vi "Handle Command.vi"(8 "error in":errorcluster, 10 "Change Laser Frequency in":refnum<class "Change Laser Frequency.lvclass">, 11 "Object In":refnum<class>) -> (0 "error out":errorcluster, 1 "Command Successful?":bool, 2 "Change Laser Frequency out":refnum<class "Change Laser Frequency.lvclass">, 3 "Object Out":refnum<class>)   [LabVIEW 2018, in "ePAS Library.lvlib" / "Change Laser Frequency.lvclass"]
doc: "Abstract method for accomplishing the execution of a command directed to an instrument object on the wire."
uses:
  Change Laser Frequency.lvclass
  Instrument/ePAS.lvclass
  C:/Users/Labview/Documents/exscalabar_server/reusable/PAS/Main/PAS.lvclass
  C:/Users/Labview/Documents/exscalabar_server/reusable/Instrument/Instrument.lvclass
  reusable/PAS/Data/Main/PAS Data.lvclass
  C:/Users/Labview/Documents/exscalabar_server/reusable/Data/Data.lvclass
  Change Laser Frequency.lvclass/Change Laser Frequency.ctl
  Instrument/ePAS.lvclass/ePAS.ctl
  reusable/Instrument/Instrument.lvclass/Instrument.ctl
  reusable/PAS/Data/Cell/PAS Cell Data.lvclass/PAS Cell Data.ctl
  reusable/PAS/Cell/PAS Cell.lvclass/PAS Cell.ctl
  reusable/PAS/Data/Cell/Write fmod.vi
  reusable/PAS/Cell/Write Mod Freq.vi
  Instrument/Accessors/Read FPGA Session.vi
  reusable/Instrument/Read ExtCom.vi
  reusable/Instrument/Read Log Session.vi
  reusable/Instrument/Read Data.vi
  reusable/Instrument/Write Data.vi
  reusable/PAS/Main/Read Cells.vi
  <vilib>/Utility/error.llb/Error Cluster From Error Code.vi
  <vilib>/rvi/errors/niLvFpgaAdjustHostInterfaceError.vi
  reusable/PAS/Data/Main/Read CellData.vi
  reusable/PAS/Data/Main/Write CellData.vi
  reusable/PAS/Main/Write Cells.vi
  reusable/PAS/Cell/PAS Cell.lvclass
  <userlib>/_Session Fwk/Session - Root.lvclass
  reusable/Data/Data.lvclass
  <vilib>/rvi/interface/nirviReadWriteControl/nirviReadWriteControl.xnode
  FPGA/R FPGA Ref.ctl
  FPGA Bitfiles/FPGAServer.lvbitx
  reusable/PAS/Data/Cell/PAS Cell Data.lvclass
  FPGA/Session/Exscalabar FPGA.lvclass
  ePAS Library.lvlib
  reusable/Session APIs/Session Log/System Log.lvclass
  NiFpgaLv.dll
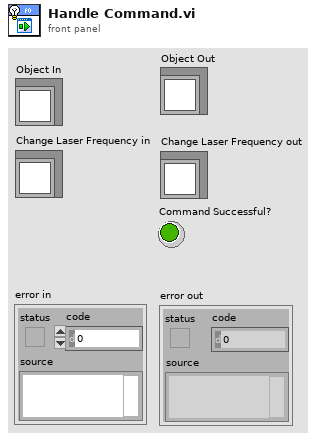
[diagram p1: front panel]
types:
  T1 = typedef "Session - Root.lvclass/Session Handle.ctl" = refnum<data-value>
  T2 = typedef "ePAS Library.lvlib/R FPGA Ref.ctl" = refnum<k20>
  T3 = cluster{"f0":fxp<+,32,0>, "Scale":fxp<+,32,0>, "Offset":i16, "Mod":enum8{"Sine", "Square"}}
  T4 = cluster{"f0":fxp<+,32,0>, "Scale":fxp<+,32,0>, "Offset":i16, "Mod":enum8{"Sine", "Square"}}[]
  T5 = cluster{"tag":string, "section":string, "data":variant}
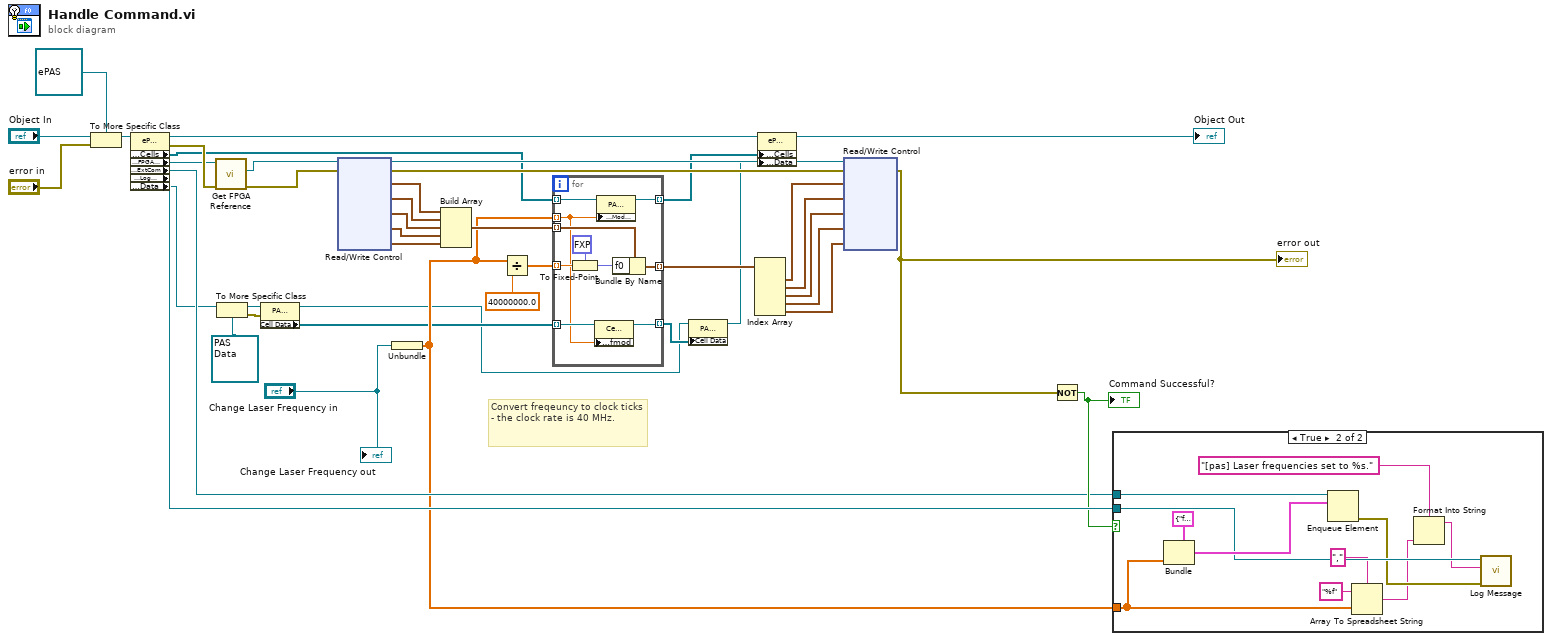
[diagram p0: block diagram]
diagram:
  # "Convert freqeuncy to clock ticks - the clock rate is 40 MHz."
  n1 = To More Specific Class(target class=refnum<class "ePAS.lvclass"> refnum ("ePAS"), reference="Object In", error in="error in") -> (specific class reference=w18:refnum<class "ePAS.lvclass">)  [unwired: 1 out]
  n2 = property class="ePAS"(reference=w18) -> (reference out=w11:refnum<class "ePAS.lvclass">, error out=w17:errorcluster, "Data Access:Cells"=w13:refnum<class "PAS Cell.lvclass">[], "Accessors:FPGA Session"=w14:T1, "Accessors:ExtCom"=w19:refnum<queue>, "Accessors:Log Session"=w21:T1, "Accessors:Data"=w8:refnum<class "Data.lvclass">)  [unwired: 1 in]
  n3 = call "Get FPGA Reference.vi"("error in"=w17, "Session In"=w14) -> ("error out"=w24:errorcluster, "Ex FPGA Ref"=w40:T2)  [unwired: 7 in, 1 out]
  n4 = To More Specific Class(target class=refnum<class "PAS Data.lvclass"> refnum ("PAS Library.lvlib:PAS Data"), reference=w8) -> (specific class reference=w5:refnum<class "PAS Data.lvclass">, error out=w6:errorcluster)  [unwired: 1 in]
  n5 = property class="PAS Data"(reference=w5, error in=w6) -> (reference out=w2:refnum<class "PAS Data.lvclass">, "Cell Data"=w4:refnum<class "PAS Cell Data.lvclass">[])  [unwired: 1 out]
  n6 = xnode "Read/Write Control"("FPGA VI Reference In"=w40, "error in"=w24) -> ("FPGA VI Reference Out"=w33:T2, "error out"=w32:errorcluster, "Cell 1"=w39:T3, "Cell 2"=w38:T3, "Cell 3"=w37:T3, "Cell 4"=w36:T3, "Cell 5"=w35:T3)
  n7 = Unbundle("Change Laser Frequency in") -> (w12:sgl[])
  n8 = Build Array(w39, w38, w37, w36, w35) -> (w34:T4)
  n9 = Divide(x=w12, y=sgl 40000000.0) -> (x/y=w15:sgl[])
  n10 = for {
    tunnel: w34 -> [w52] mode=indexing
    tunnel: [w49] -> w31 mode=indexing
    tunnel: w15 -> [w48] mode=indexing
    tunnel: w13 -> [w47] mode=indexing
    tunnel: w12 -> [w44] mode=indexing
    tunnel: [w46] -> w9 mode=indexing
    tunnel: w4 -> [w45] mode=indexing
    tunnel: [w43] -> w3 mode=indexing
    n11 = To Fixed-Point(fixed-point type=fxp<+,32,0> 0.0 ("f0"), number=w48) -> (fixed-point=w50:fxp<+,32,0>)
    n12 = property class="Cell Data"(reference=w45, "Accessors:fmod"=w44) -> (reference out=w43:refnum<class "PAS Cell Data.lvclass">)  [unwired: 1 in, 1 out]
    n13 = property class="PAS Cell"(reference=w47, "Accessors:Mod Freq"=w44) -> (reference out=w46:refnum<class "PAS Cell.lvclass">)  [unwired: 1 in, 1 out]
    n14 = Bundle By Name(cluster=w52, "f0"=w50) -> (w49:T3)
  }
  n15 = property class="PAS Data"(reference=w2, "Cell Data"=w3) -> (reference out=w1:refnum<class "PAS Data.lvclass">)  [unwired: 1 in, 1 out]
  n16 = Index Array(array=w31) -> (element #1=w30:T3, element #2=w29:T3, element #3=w28:T3, element #4=w27:T3, element #5=w26:T3)  [unwired: 5 in]
  n17 = property class="ePAS"(reference=w11, "Data Access:Cells"=w9, "Accessors:Data"=w1) -> (reference out=→"Object Out":refnum<class "ePAS.lvclass">)  [unwired: 1 in, 1 out]
  n18 = xnode "Read/Write Control"("FPGA VI Reference In"=w33, "error in"=w32, "Cell 1"=w30, "Cell 2"=w29, "Cell 3"=w28, "Cell 4"=w27, "Cell 5"=w26) -> ("error out"=w23:errorcluster)  [unwired: 1 out]
  "error out" <- w23
  n19 = Not(x=w23) -> (.not. x?=w20:bool)
  "Command Successful?" <- w20
  n20 = case shown="True" w20 {
    tunnel: w19 -> [_ w63]
    tunnel: w12 -> [_ w56]
    tunnel: w21 -> [_ w60]
    frame False {
    }
    frame True {
      n21 = Bundle(cluster=T5 {"tag"="f0", "section"="pas.las", "data"=variant} ("element"), "data"=w56) -> (w61:T5)  [unwired: 2 in]
      n22 = Enqueue Element(queue=w63, element=w61) -> (error out=w57:errorcluster)  [unwired: 2 in, 2 out]
      n23 = Array To Spreadsheet String(delimiter (Tab)=",", array=w56, 3:"%f" ("format string")) -> (spreadsheet string=w54:string)
      n24 = Format Into String(format string="[pas] Laser frequencies set to %s.", w54) -> (resulting string=w58:string)  [unwired: 2 in, 1 out]
      n25 = call "Log Message.vi"("error in"=w57, "MSG In"=w58, "session in"=w60) -> ()  [unwired: 7 in, 2 out]
    }
  }
  "Change Laser Frequency out" <- "Change Laser Frequency in"
